vi "CoreChem_Interface_v1.vi"() -> ()   [LabVIEW 2014]
panel:
  in  "Tab Control":T1(tab)
  in  "OK Button":bool
  in  "SO2":bool
  in  "CO":bool
  in  "FGGA":bool
  in  "2B Ozone":bool
  in  "TECO Ozone":bool
  out "Zero":dbl
  out "Sensitivity":dbl
  out "Sig":dbl
  out "Conc":dbl
  in  "Plasma Lamp":bool
  in  "CO VACUUM":bool
  in  "Prepare Gases":bool
  in  "CO checks":bool
  out "CO preflight Des 1":string="CO Ground Preflight Checks\n\n1.\n\n\n\n2. Start CO Vacuum. NB: If there is problem with the software control, use manual override switch [up] on CALDECK front panel\n\n\n\n\n\n3. Check Plasma Lamp switch is down\n    Make AL5002 CB\n\n4. CO Checks\n    Lamp Flow Controller ~ 40 ml/min\n    Monochromater Flow Controller ~ 30 ml/min\n    Fluorescence Cell Pressure ~ 7.5 Torr\n\n5. Switch Plasma Lamp at the front panel UP\n   \n     \n\n"
  out "Press? F":dbl
  out "Temp? F":dbl
  out "Temp? M":dbl
  out "Temp? L":dbl
  out "Monochromater Flow Controller":dbl
  out "Lamp Flow Controller":dbl
  out "CO pump":bool
  out "Press? M":dbl
  out "Fluorescence Cell Pressure":dbl
  out "CO CAL":bool
  in  "Show cal record":bool
  in  "CALIBRATION":bool
  out "CO2 Deliv":dbl(slide) scale=0.0..5.0
  out "Std\nContent":dbl(slide) scale=0.0..250.0
  out "N2\nContent":dbl(slide) scale=0.0..250.0
  out "CO2\nContent":dbl(slide) scale=0.0..250.0
  out "error out":errorcluster
  out "Boolean 19":bool
  out "Boolean 18":bool
  out "Boolean 17":bool
  out "Boolean 16":bool
  out "Boolean 15":bool
  out "Boolean 14":bool
  out "Boolean 13":bool
  out "Boolean 12":bool
  out "Boolean 11":bool
  out "Boolean 10":bool
  out "Boolean 9":bool
  out "Boolean 8":bool
  out "Boolean 7":bool
  out "Boolean 6":bool
  out "Boolean 5":bool
  out "Boolean 4":bool
  out "Boolean 3":bool
  out "Boolean 2":bool
  out "Boolean":bool
  in  "LCD check 4":bool
  in  "LCD check 3":bool
  in  "LCD check 2":bool
  in  "OK Button 2":bool
  out "Value Read":string
  out "FGGA preflight Des 5":string="Caldeck Mass Flow Control"
  out "Purge Time Remain (sec)":u32
  in  "Low Flush":bool
  in  "Target Flush":bool
  in  "High Flush":bool
  out "Calibration Time \nRemain (sec)":u32
  out "FGGA preflight Des 3":string="FGGA CAL Gas Purge\n\nFor each cylinder in gas stowage, check that,\n\n1. V1 Closed\n    V3 Closed\n    V4 Make sure arrow positioned downwards (i.e. flow points to gas line)\n\n2. V3 Open (turn anti-clockwise)\n\n3. Use the button on the right according to the operating cylinder to flush the line. Monitor the MFC flow rate to make sure the reading decreases from 3 to zero. (ie fully flushed). Pressure content & delivery gauges should also read zero.\n\n4. V3 Close (turn clockwise)\n\n5. V1 Open / Close quickly\n         Check delivery pressure gauge is ~ 40 PSI (Use V2         to increase if necessary)\n\n6. Repeat steps 2 to 5 three times\n\n7. V3 Close (turn clockwise)\n\n8. V1 Open, check V2 ~ 40 PSIG\n\n9. V3 Open - System is ready"
  in  "LCD check":bool
  out "FGGA preflight Des 2":string="4. Check Time Synchronisation\n\n5. Check CO2 & CH4 values\n\n\n6. Stow LCD monitor and keybaord"
  out "FGGA preflight Des 1":string="FGGA Ground Preflight Checks\n\n1. Switch FGGA pump ON\n\n2. Check cavity pressure ~50 Torr\n\n3. Switch FGGA pump OFF"
  in  "cavity press check 2":bool
  in  "FGGA pump on check 2":bool
  out "H2O":dbl
  out "CH4":dbl
  out "CO2":dbl
  in  "FGGA pump off check":bool
  in  "cavity press check":bool
  in  "FGGA pump on check":bool
  out "Cavity Pressure":dbl
  in  "FGGA pump":bool
  out "Flush Time \nRemain (sec)":u32
  out "Alicat MFC":dbl
  out "V1":bool
  out "V4":bool
  out "V2":bool
  out "V3":bool
  in  "Target Cal":bool
  in  "Low Cal":bool
  in  "High Cal":bool
  out "FGGA preflight Des 4":string="Inflight Calibration\n\nHigh\n\nLow\n\nTarget"
  in  "SLPM Value to be set":dbl=1.5
  # "High             Target         Low"
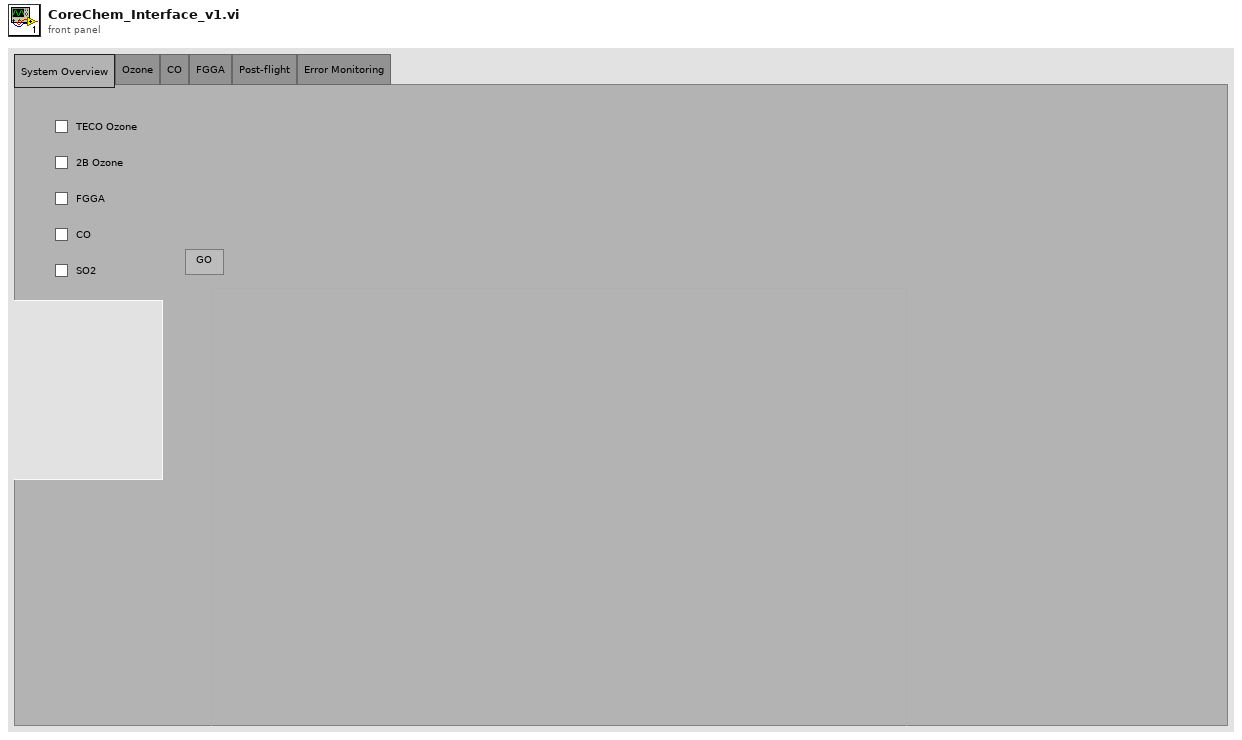
[diagram p1: front panel]
types:
  T1 = enum32{"System Overview", "Ozone", "CO", "FGGA", "Post-flight", "Error Monitoring"}
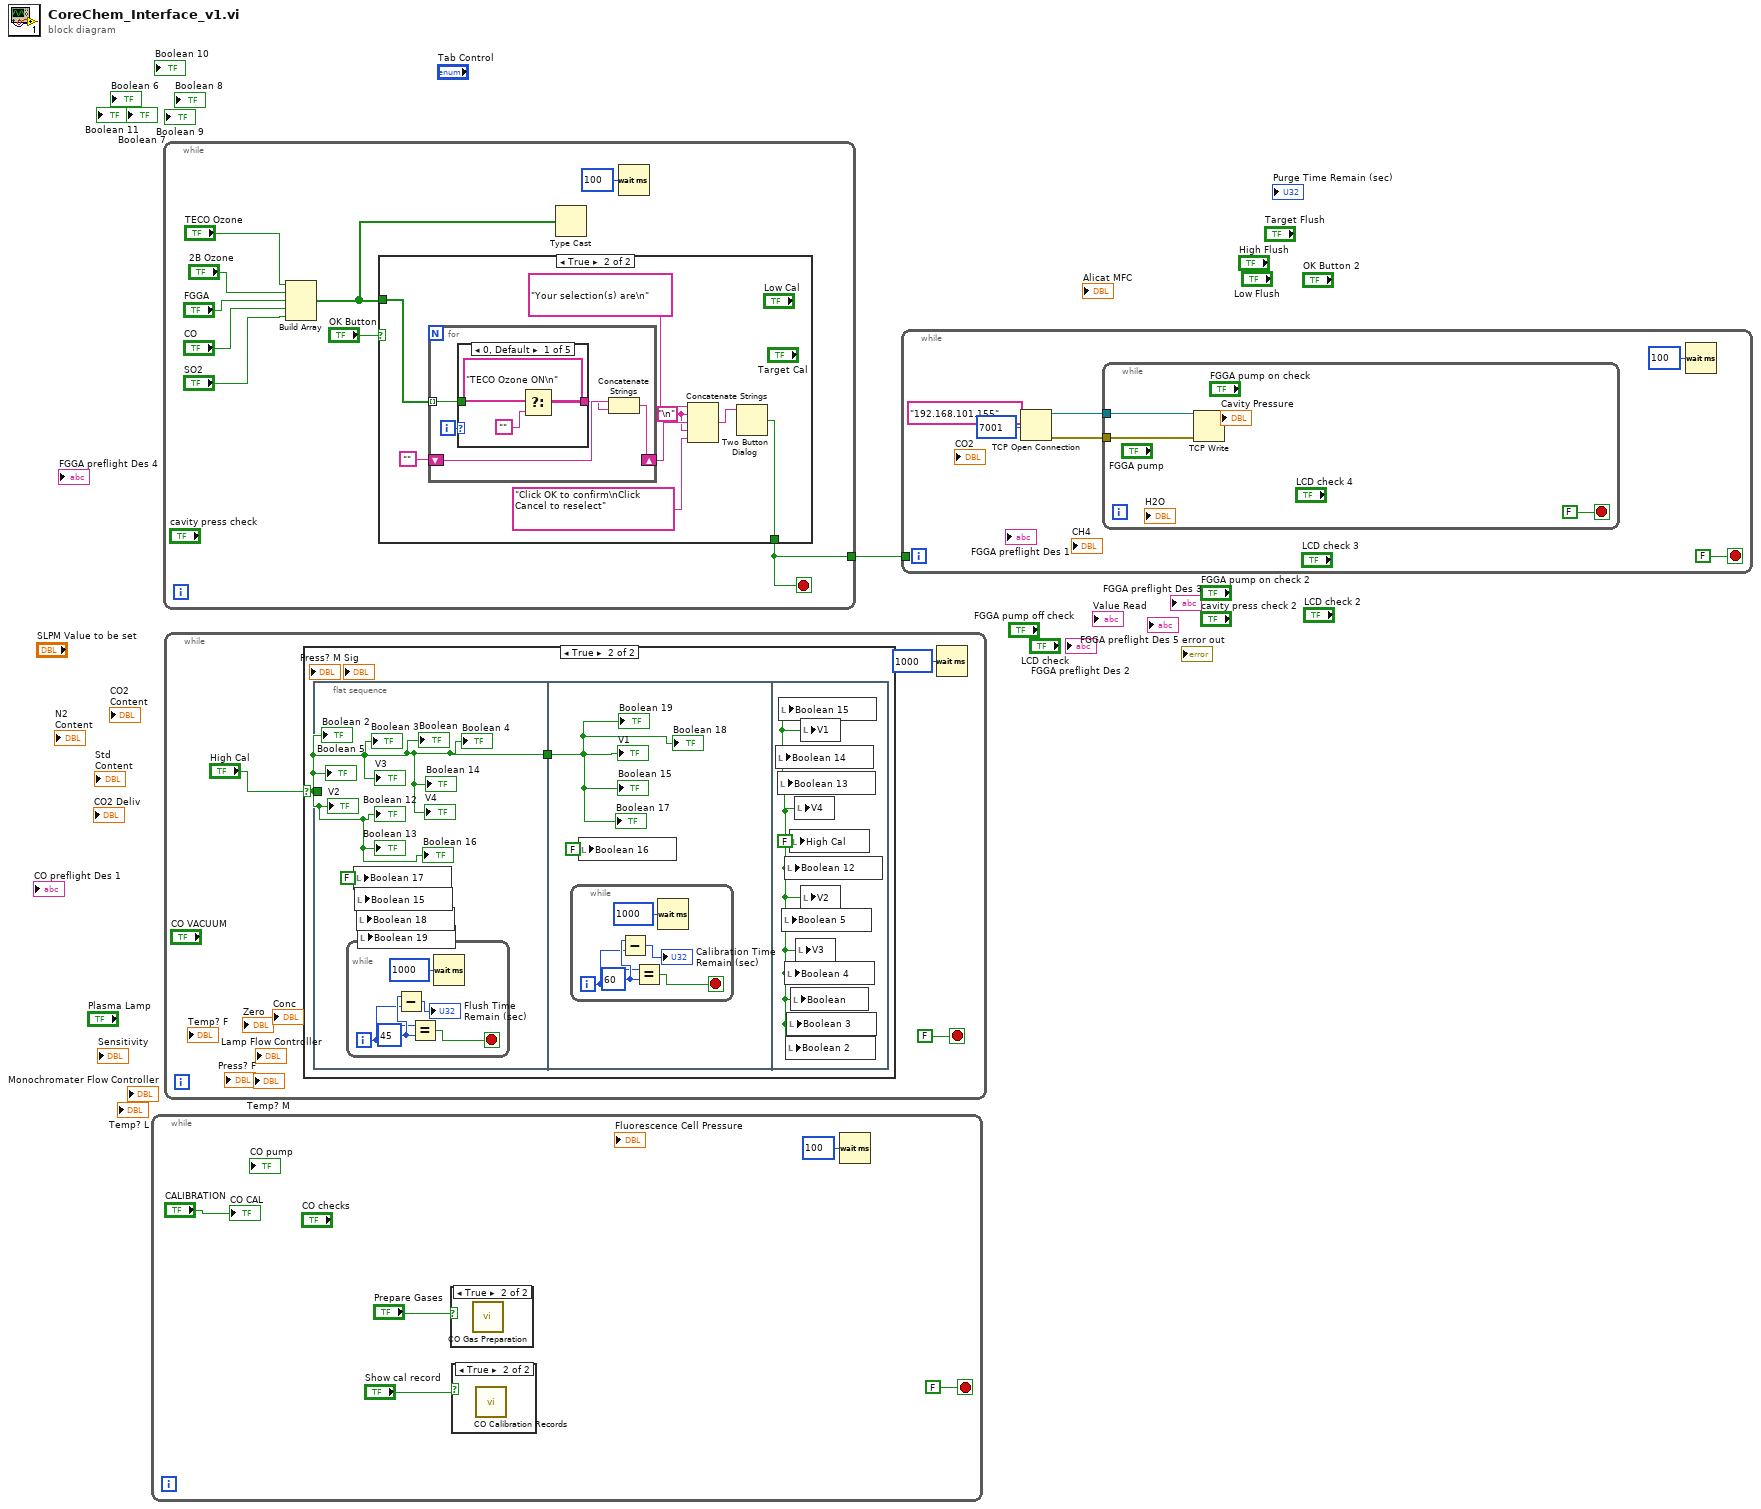
[diagram p0: block diagram]
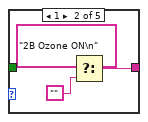
[diagram p6: hidden frame]
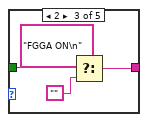
[diagram p7: hidden frame]
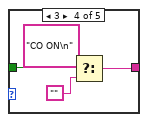
[diagram p8: hidden frame]
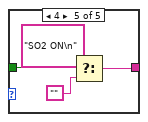
[diagram p9: hidden frame]
diagram:
  n1 = while {
    stop <- FALSE stop-if-true
    n2 = case shown="True" "Prepare Gases" {
      frame False {
      }
      frame True {
        n3 = call "CO Gas Preparation.vi"() -> ()  [unwired: 12 in]
      }
    }
    n4 = case shown="True" "Show cal record" {
      frame False {
      }
      frame True {
        n5 = call "CO Calibration Records.vi"() -> ()  [unwired: 12 in]
      }
    }
    n6 = Wait (ms)(milliseconds to wait=u32 100) -> ()  [unwired: 1 out]
    "CO CAL" <- "CALIBRATION"
  }
  n7 = while {
    tunnel: [w9] -> w1
    stop <- w9 stop-if-true
    n8 = Build Array("TECO Ozone", "2B Ozone", "FGGA", "CO", "SO2") -> (w7:bool[])
    n9 = case shown="True" "OK Button" {
      selector: "OK Button" -> [w16 _]
      tunnel: w7 -> [_ w24]
      tunnel: [w16 w18] -> w9
      frame False {
      }
      frame True {
        w17 = "\n"
        n10 = for {
          tunnel: w24 -> [w28] mode=indexing
          shift-right: [w27] -> w22
          shift-left: "" -> [w26]
          i -> [w29]
          n11 = case shown="0, Default" w29 {
            tunnel: w28 -> [w33 w37 w41 w45 w49]
            tunnel: [w30 w34 w38 w42 w46] -> w25
            frame 0, Default {
              n12 = Select(t="TECO Ozone ON\n", s=w33, f="") -> (s? t:f=w30:string)
            }
            frame 1 {
              n13 = Select(t="2B Ozone ON\n", s=w37, f="") -> (s? t:f=w34:string)
            }
            frame 2 {
              n14 = Select(t="FGGA ON\n", s=w41, f="") -> (s? t:f=w38:string)
            }
            frame 3 {
              n15 = Select(t="CO ON\n", s=w45, f="") -> (s? t:f=w42:string)
            }
            frame 4 {
              n16 = Select(t="SO2 ON\n", s=w49, f="") -> (s? t:f=w46:string)
            }
          }
          n17 = Concatenate Strings(w26, w25) -> (w27:string)
        }
        n18 = Concatenate Strings("Your selection(s) are\n" ("string"), w17, w22, w17, "Click OK to confirm\nClick Cancel to reselect" ("string")) -> (w19:string)
        n19 = Two Button Dialog(message=w19) -> (T button?=w18:bool)  [unwired: 2 in]
      }
    }
    n20 = Type Cast(x=w7) -> ()  [unwired: 1 in, 1 out]
    n21 = Wait (ms)(milliseconds to wait=u32 100) -> ()  [unwired: 1 out]
  }
  n22 = while {
    stop <- FALSE stop-if-true
    n23 = case shown="True" "High Cal" {
      selector: "High Cal" -> [_ w54]
      frame False {
      }
      frame True {
        n24 = flat-sequence {
          tunnel: w54 -> [w56]
          tunnel: [w56] -> w53
          tunnel: w53 -> [w62]
          frame #0 {
            w55 = FALSE ("Boolean 17")
            n25 = while {
              i -> [w58]
              stop <- w61 stop-if-true
              w59 = 45 ("y")
              n26 = Subtract(x=w59, y=w58) -> (x-y=→"Flush Time \nRemain (sec)":i32)
              n27 = Equal?(x=w58, y=w59) -> (x = y?=w61:bool)
              n28 = Wait (ms)(milliseconds to wait=u32 1000) -> ()  [unwired: 1 out]
            }
            n29 = local write "Boolean 17"(w55) -> ()
            n30 = local write "Boolean 15"(w55) -> ()
            n31 = local write "Boolean 18"(w55) -> ()
            n32 = local write "Boolean 19"(w55) -> ()
            "Boolean 3" <- w56
            "Boolean" <- w56
            "Boolean 4" <- w56
            "V3" <- w56
            "Boolean 5" <- w56
            "V2" <- w56
            "Boolean 2" <- w56
            "Boolean 12" <- w56
            "Boolean 13" <- w56
            "Boolean 14" <- w56
            "Boolean 16" <- w56
            "V4" <- w56
          }
          frame #1 {
            n33 = while {
              i -> [w65]
              stop <- w68 stop-if-true
              w66 = 60 ("y")
              n34 = Subtract(x=w66, y=w65) -> (x-y=→"Calibration Time \nRemain (sec)":i32)
              n35 = Equal?(x=w65, y=w66) -> (x = y?=w68:bool)
              n36 = Wait (ms)(milliseconds to wait=u32 1000) -> ()  [unwired: 1 out]
            }
            n37 = local write "Boolean 16"(FALSE ("Boolean 16")) -> ()
            "V1" <- w62
            "Boolean 15" <- w62
            "Boolean 17" <- w62
            "Boolean 19" <- w62
            "Boolean 18" <- w62
          }
          frame #2 {
            w69 = FALSE ("High Cal")
            n38 = local write "Boolean 14"(w69) -> ()
            n39 = local write "Boolean 13"(w69) -> ()
            n40 = local write "Boolean 15"(w69) -> ()
            n41 = local write "Boolean 5"(w69) -> ()
            n42 = local write "Boolean 12"(w69) -> ()
            n43 = local write "Boolean 4"(w69) -> ()
            n44 = local write "Boolean 2"(w69) -> ()
            n45 = local write "Boolean 3"(w69) -> ()
            n46 = local write "High Cal"(w69) -> ()
            n47 = local write "Boolean"(w69) -> ()
            n48 = local write "V4"(w69) -> ()
            n49 = local write "V3"(w69) -> ()
            n50 = local write "V1"(w69) -> ()
            n51 = local write "V2"(w69) -> ()
          }
        }
      }
    }
    n52 = Wait (ms)(milliseconds to wait=u32 1000) -> ()  [unwired: 1 out]
  }
  n53 = while {
    tunnel: w1 -> [_]
    stop <- FALSE stop-if-true
    n54 = TCP Open Connection(address="192.168.101.155", remote port or service name=u16 7001) -> (connection ID=w74:refnum<k5>, error out=w73:errorcluster)  [unwired: 3 in]
    n55 = while {
      tunnel: w74 -> [w78]
      tunnel: w73 -> [w77]
      stop <- FALSE stop-if-true
      n56 = TCP Write(connection ID=w78, error in (no error)=w77) -> ()  [unwired: 2 in, 3 out]
    }
    n57 = Wait (ms)(milliseconds to wait=u32 100) -> ()  [unwired: 1 out]
  }
